vi "电导率电极校准.vi"() -> ()   [LabVIEW 2016, in "斯坦道多参数.lvlib"]
uses:
  <vilib>/Utility/miscctls.llb/LVPointTypeDef.ctl
  <vilib>/Analysis/NI_AALBase.lvlib
panel:
  out "滤波设定":dbl
  in  "刷新按钮":bool
  out "第二点信号值":dbl
  out "第一点信号值":dbl
  out "通讯状态":string
  out "盐度":dbl caption="盐度测量值" format="%#.2f"
  out "温度":dbl format="%#.2f"
  out "当前信号值":dbl caption="信号值" format="%#.2f"
  in  "校准停止":bool
  in  "校准启动":bool
  out "波形图表":sgl(graph) caption="历史曲线"
  out "第二点校准值":dbl
  out "第一点校准值":dbl
  in  "校准模式":u16(ring)=1 items=["两点校准", "单点校准"]
  out "提示":string
  out "最小值":sgl format="%#.2f"
  out "最大值":sgl format="%#.2f"
  out "mean":dbl caption="均值" format="%#.2f"
  out "standard deviation":dbl caption="标准差" format="%#.2f"
  out "变异系数":dbl format="%#.6f"
  out "标液2":dbl
  out "标液1":dbl
  out "当前读取值":dbl caption="测量值" format="%#.2f"
  out "电极系数":dbl format="%#.6f"
  out "偏移值补偿":dbl caption="电导率偏移修正值" format="%#.2f"
  out "温度补偿系数":dbl format="%#.6f"
  # "电导率电极设定"
  # "ppt"
  # "请选择校准模式:"
  # "℃"
  # "μS/cm"
  # "cm"
  # "-1"
  # "%"
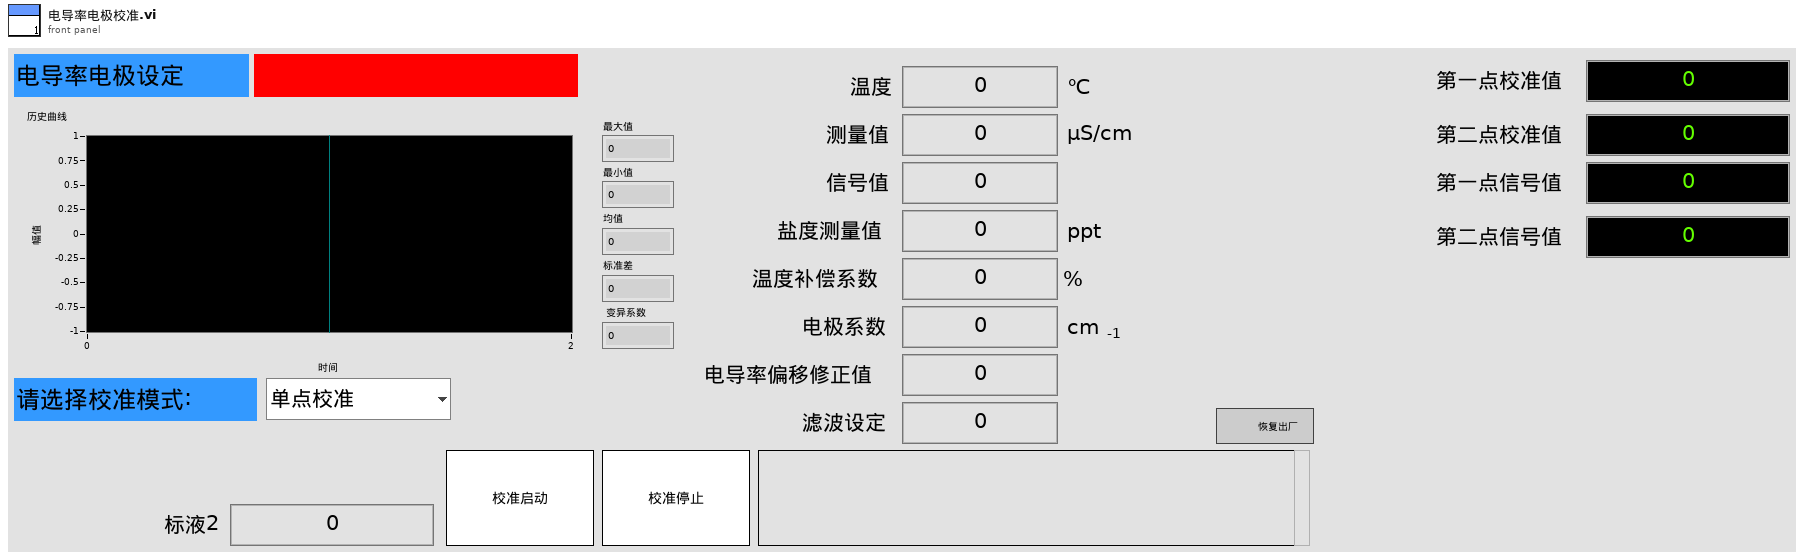
[diagram p1: front panel]
types:
  T1 = enum16{"pH", "DO", "Cond", "Turb", "ORP", "叶绿素a", "藻密度"}
  T2 = typedef "LVPointTypeDef.ctl" = cluster{"Horizontal":i16, "Vertical":i16}
  T3 = cluster{"电极状态标志":u16, "电极型号标志":u16, "电导率测量值":sgl, "温度测量值":sgl, "电导率信号值":sgl, "温度信号值":sgl, "温度补偿系数":sgl, "电导率偏移修正值":sgl, "温度偏移修正值":sgl, "手动温度补偿值":sgl, "电导率电极零点":sgl, "电导率电极斜率":sgl, "命令滤波设定":u16, "温度模式":enum16{"ATC", "MTC"}, "生产批次":u16, "电极序号":u16, "串口地址":u16, "串口波特率":enum16{"9600", "19200", "115200"}, "串口校验位":enum16{"NONE", "ODD", "EVEN"}, "串口停止位":enum16{"1bit", "2bit"}, "第一点标准值":sgl, "第二点标准值":sgl}
  T4 = enum8{"Enabled", "Disabled", "Disabled and Grayed Out"}
  T5 = cluster{"测量量程":dbl, "测量精度":dbl, "测量间隔":dbl, "消解温度":dbl, "消解时长":dbl, "空白校准时间":timestamp, "曲线截距":dbl, "曲线斜率":dbl, "测量检出限":dbl, "测量信号值":dbl, "线性相关系数":dbl, "二次多项式系数":dbl, "标样校准时间":timestamp, "稀释倍数":dbl, "三项式系数":dbl, "空白标定系数":dbl, "量程系数":dbl, "F0/ORPA":dbl, "F1/ORPB":dbl, "F2/ORPK":dbl, "F3":dbl, "F4":dbl, "F5":dbl, "F6":dbl, "F7":dbl, "X0/滴定数":dbl, "量程":dbl}
  T6 = cluster{"ph":bool, "DO":bool, "Cond":bool, "Turb":bool, "叶绿素a":bool, "藻密度":bool, "ORP":bool, "COD":bool}
  T7 = cluster{"温度测量值":sgl, "测量值":sgl, "温度偏移修正值":sgl, "信号值":sgl}
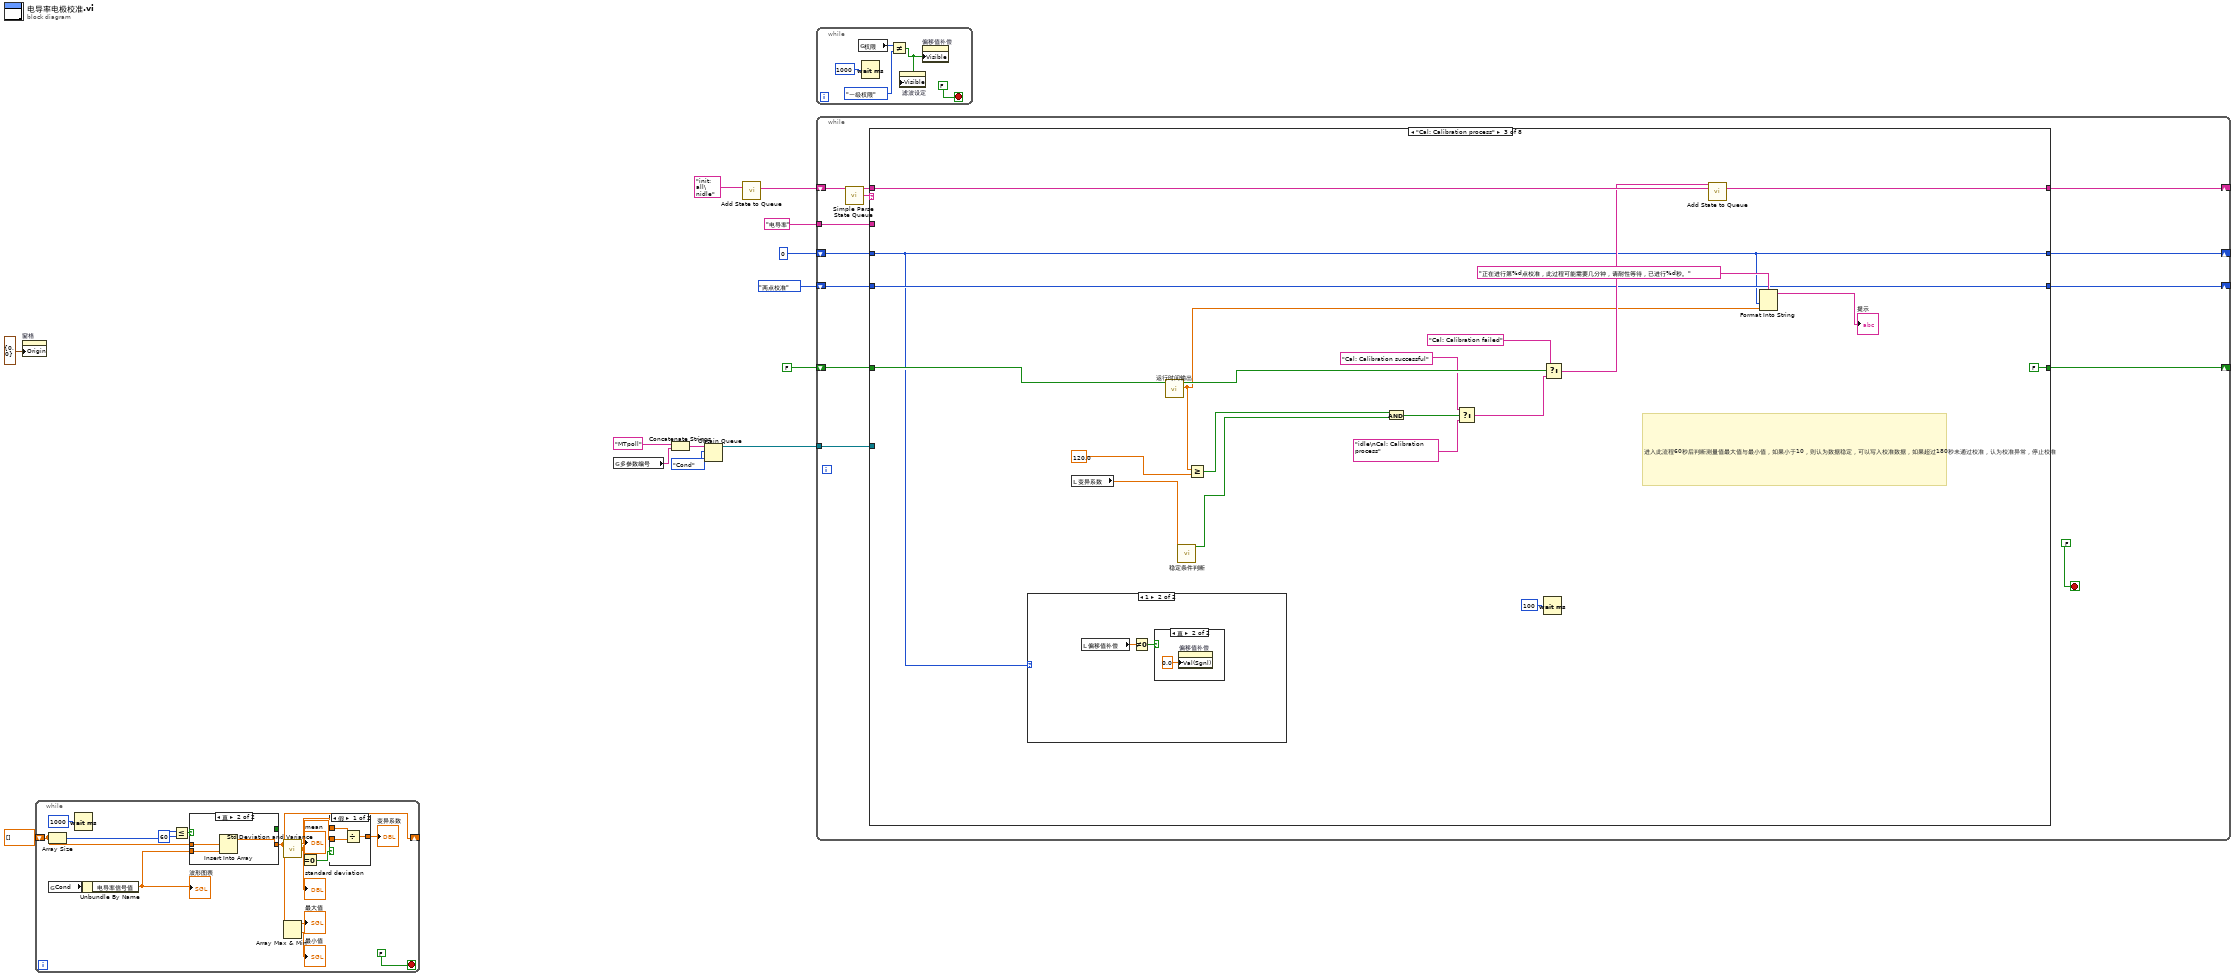
[diagram p0: block diagram]
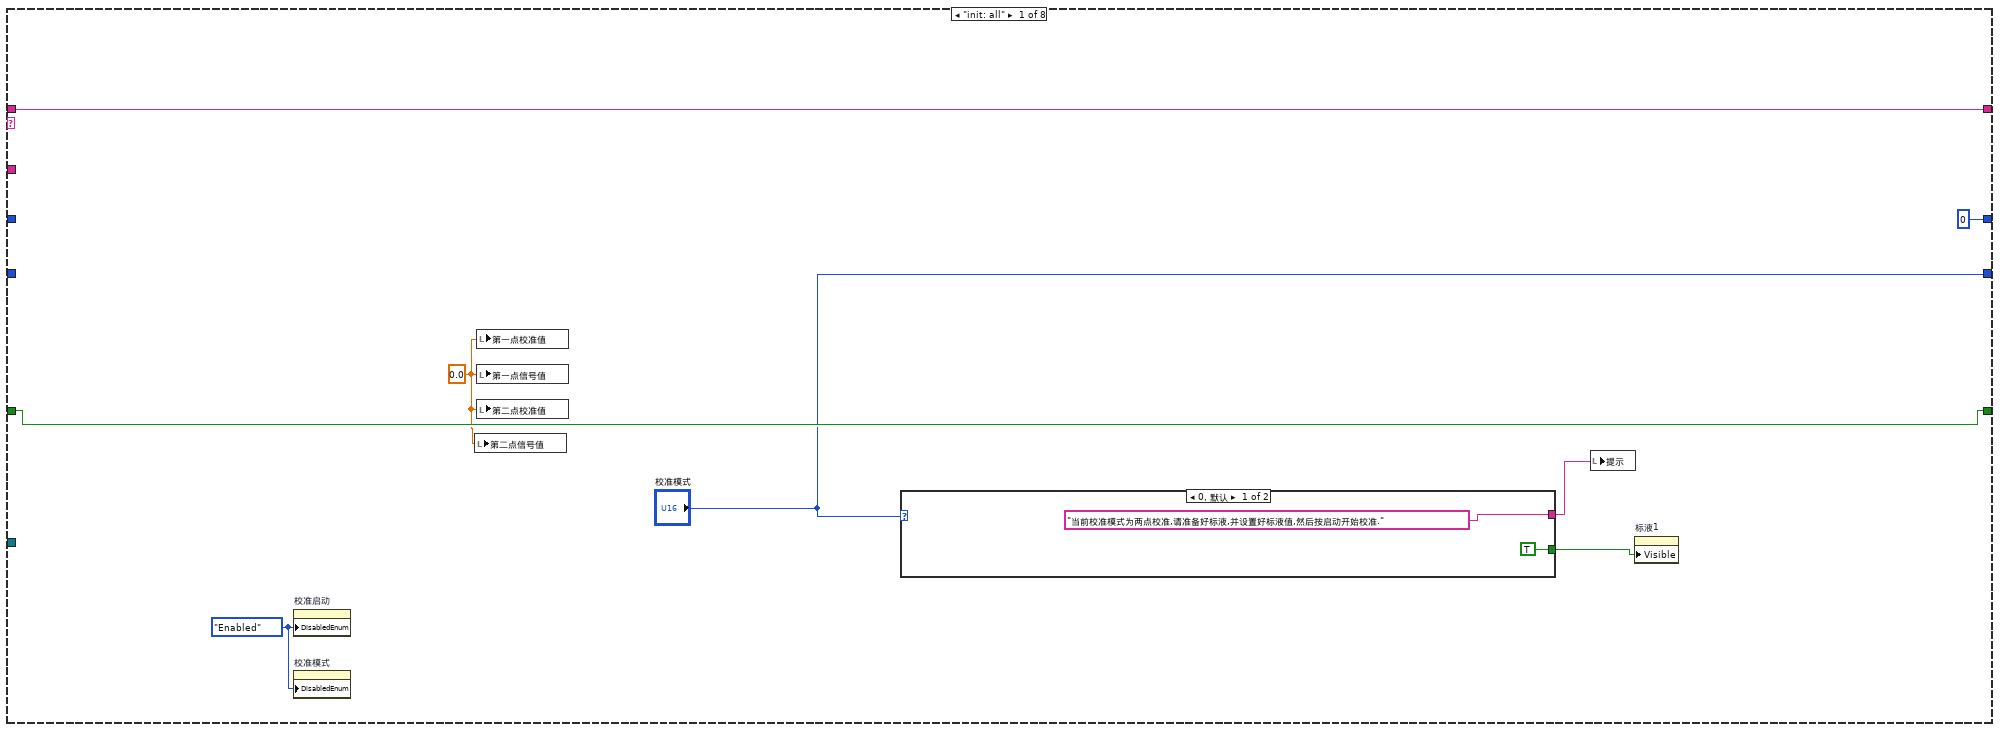
[diagram p2: hidden frame]
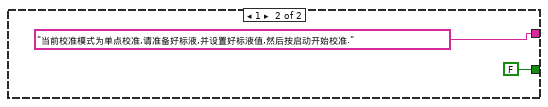
[diagram p3: hidden frame]
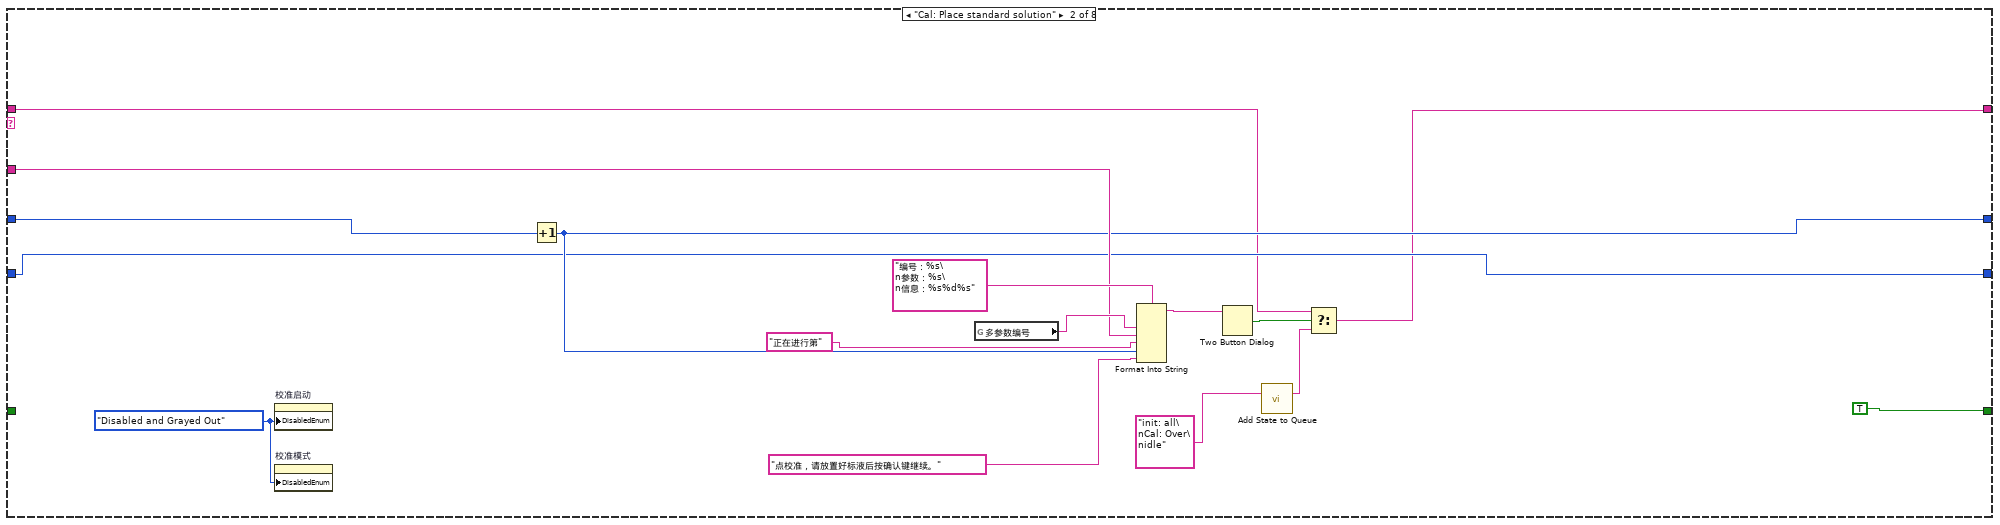
[diagram p4: hidden frame]
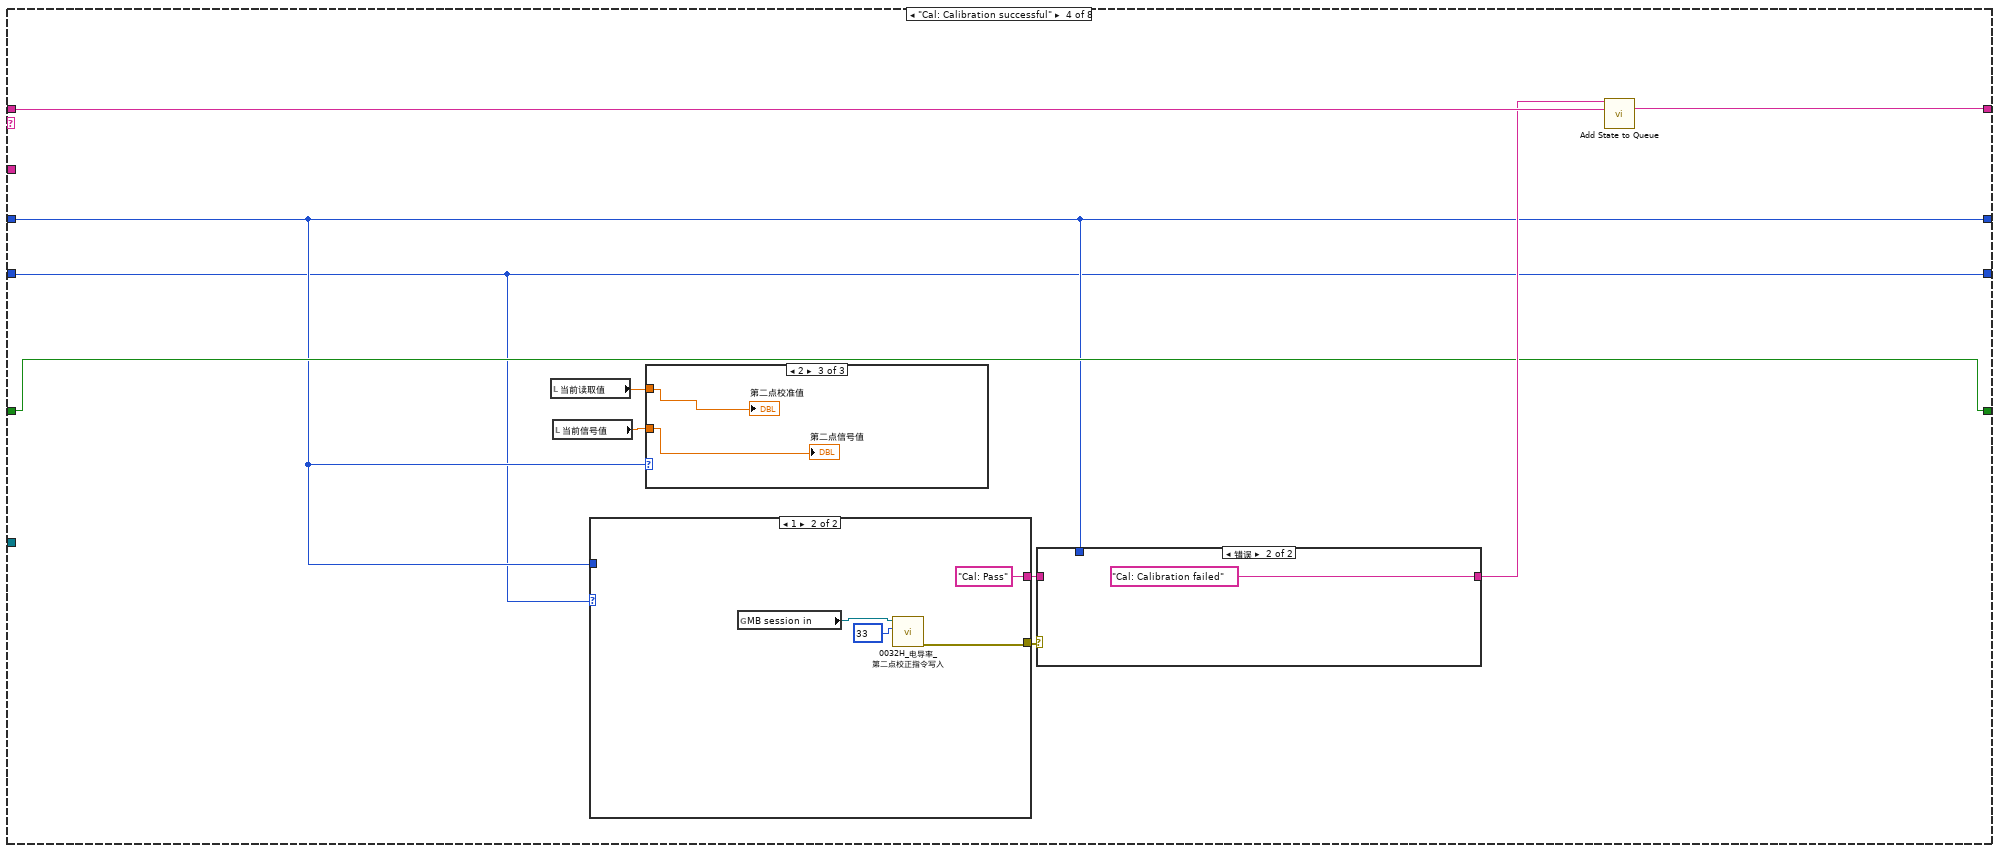
[diagram p7: hidden frame]
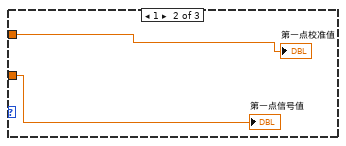
[diagram p9: hidden frame]
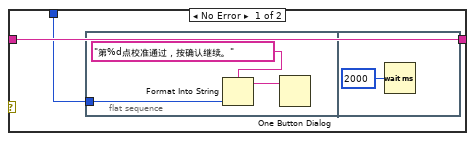
[diagram p10: hidden frame]
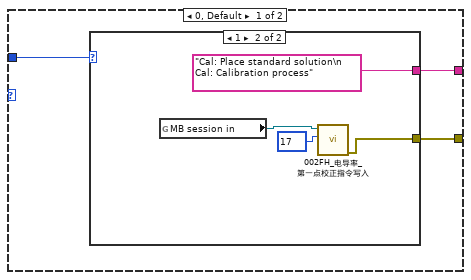
[diagram p11: hidden frame]
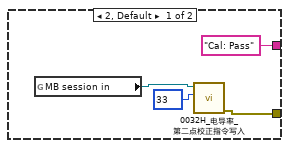
[diagram p12: hidden frame]
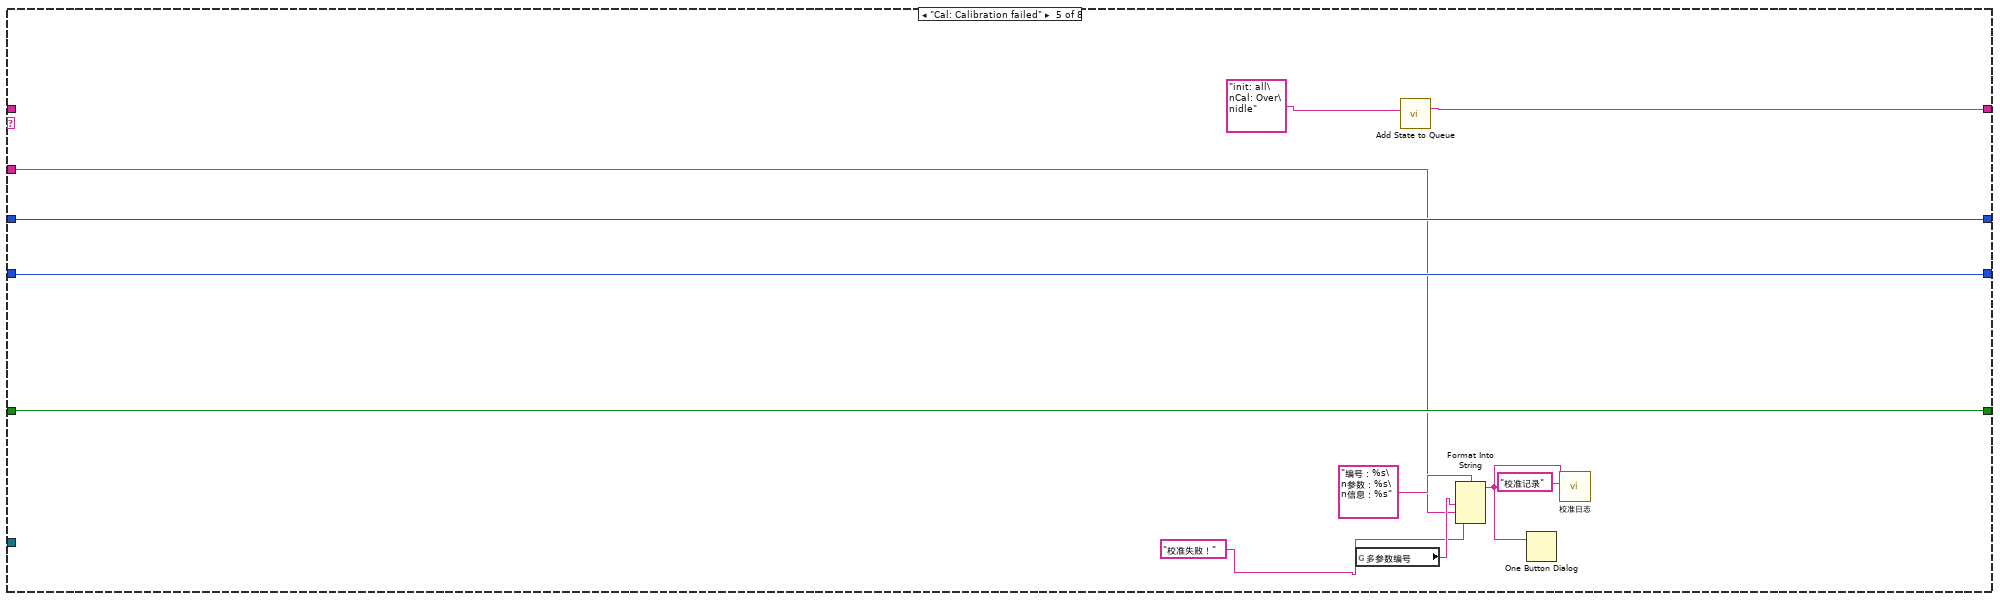
[diagram p13: hidden frame]
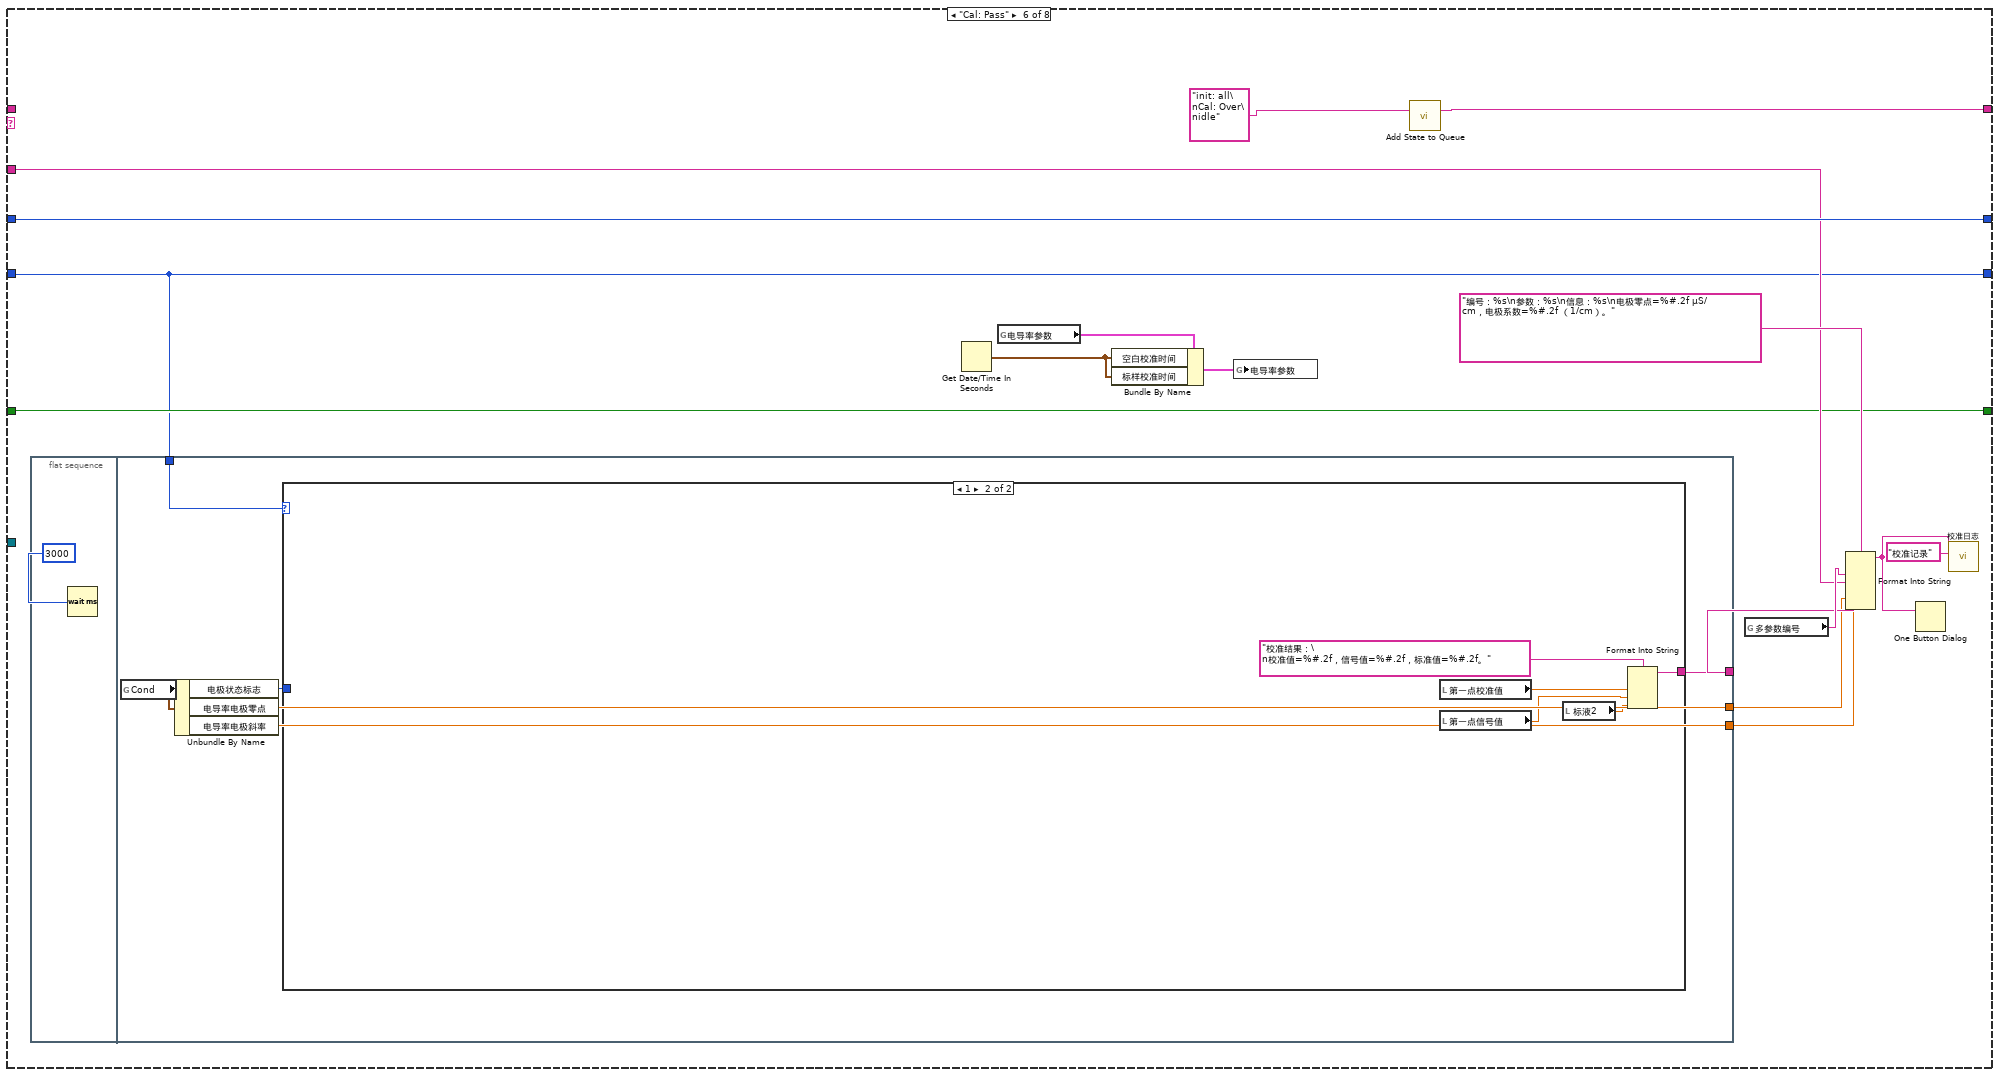
[diagram p14: hidden frame]
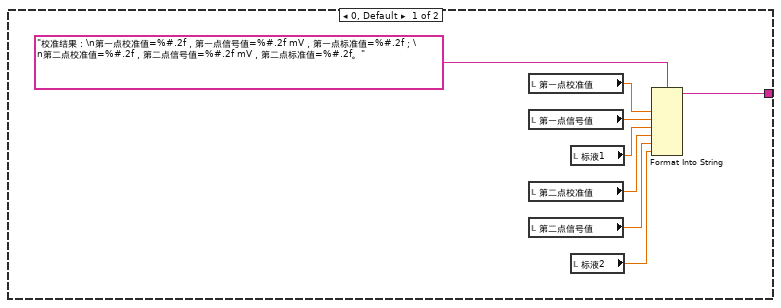
[diagram p15: hidden frame]
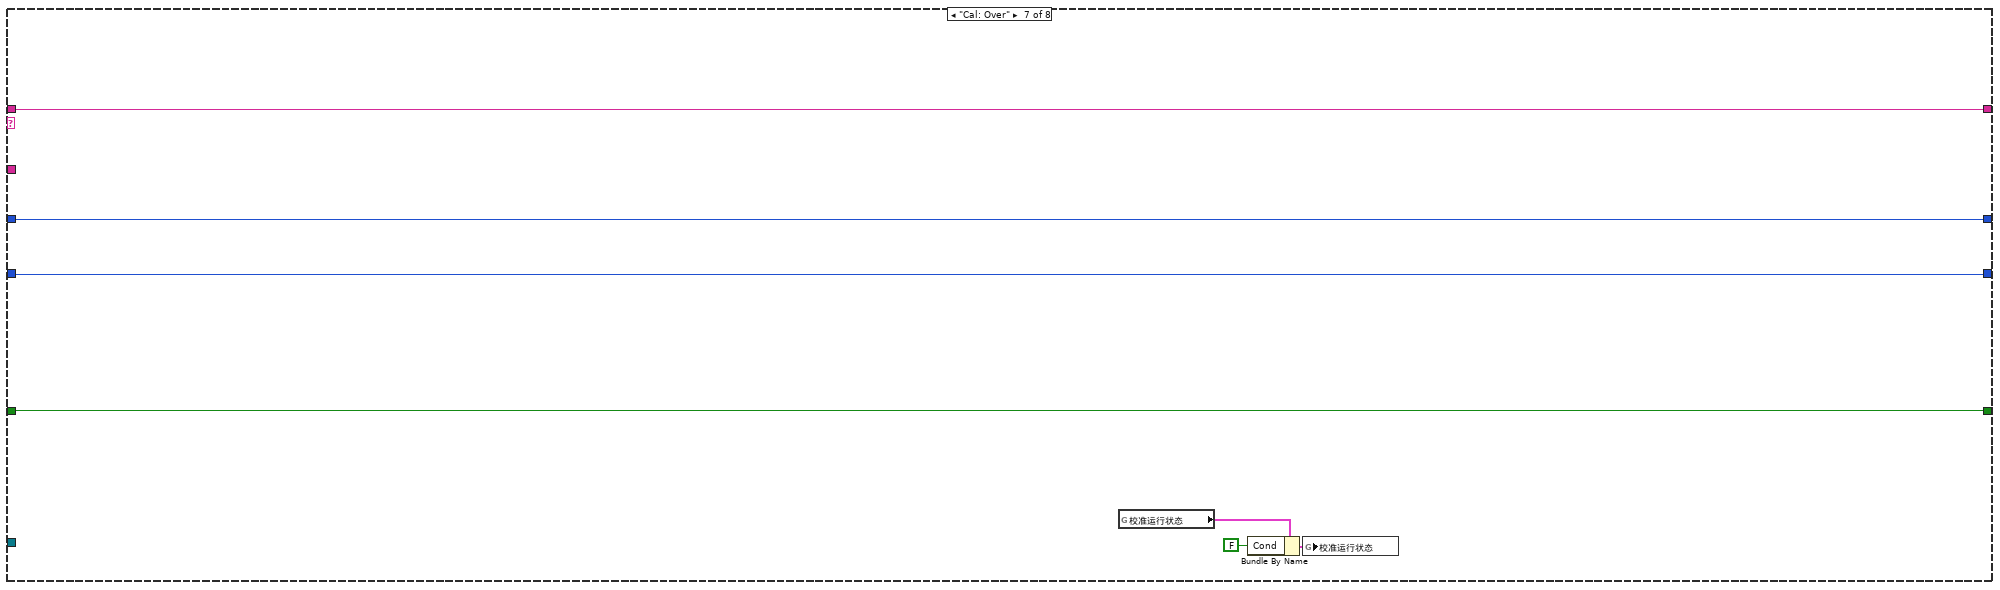
[diagram p16: hidden frame]
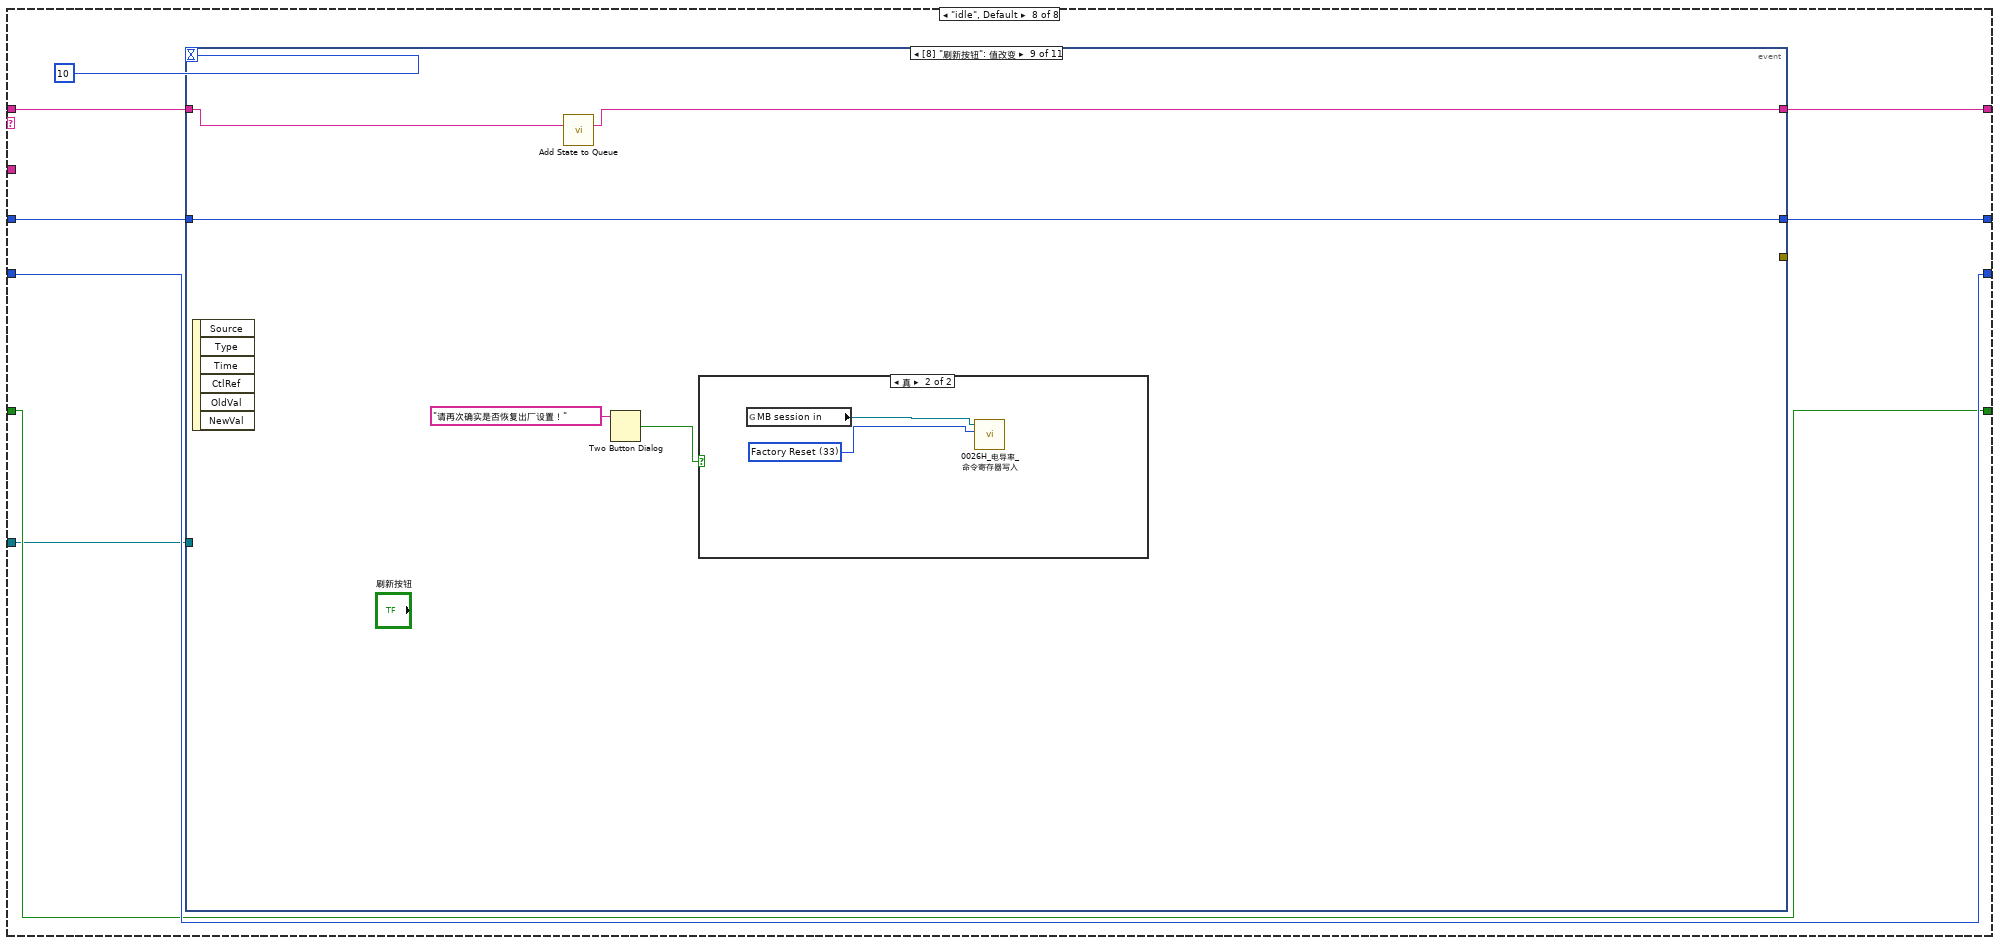
[diagram p17: hidden frame]
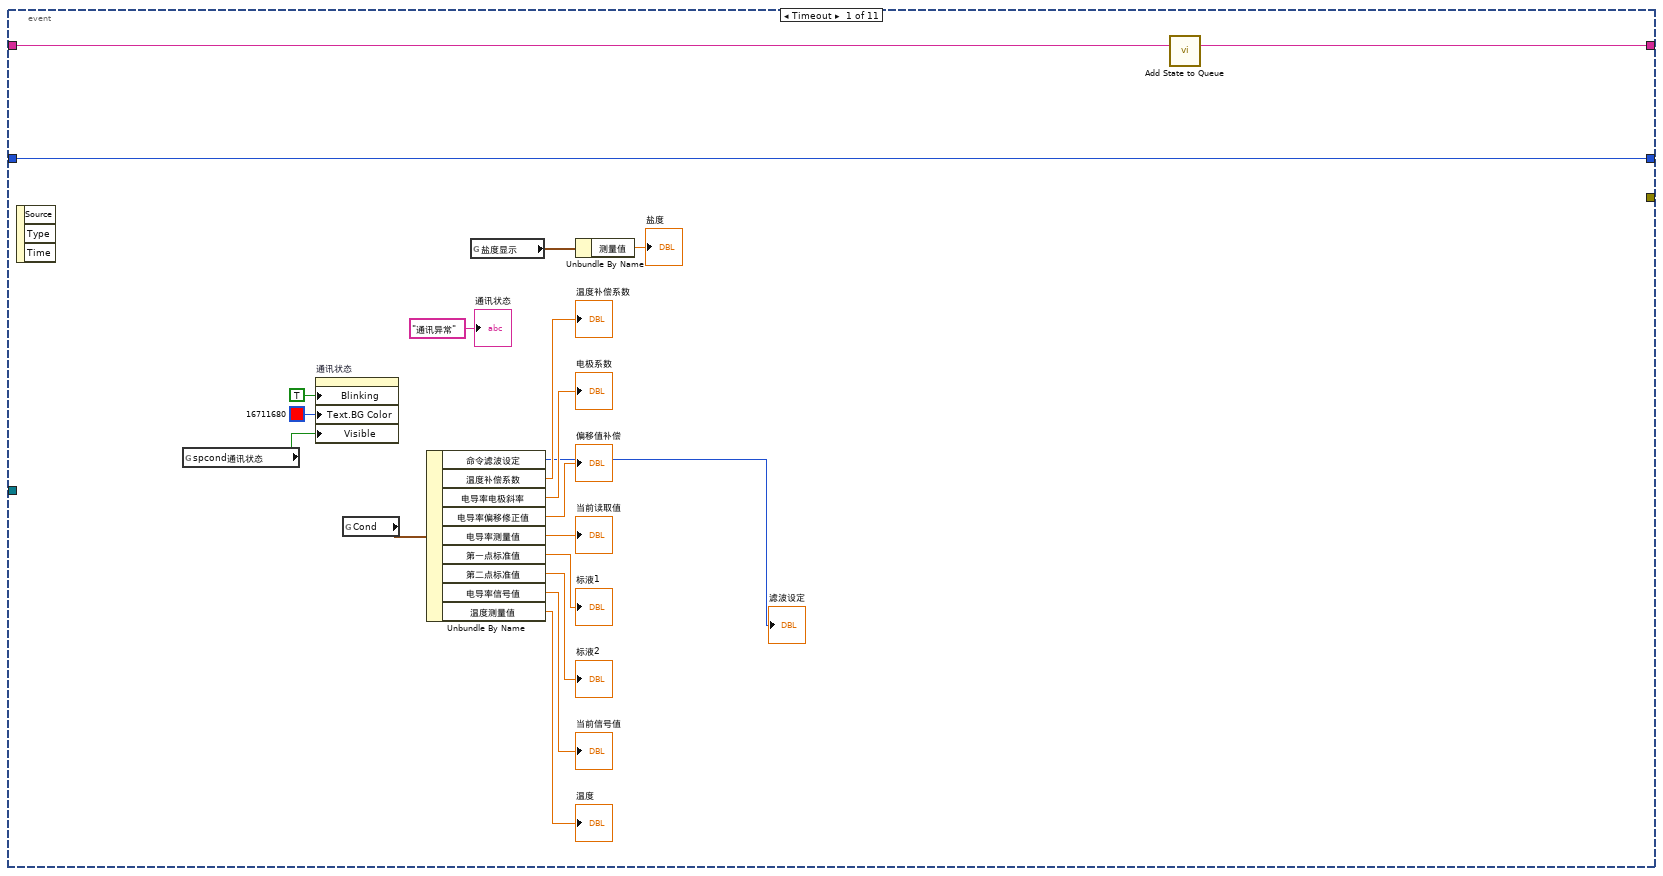
[diagram p18: hidden frame]
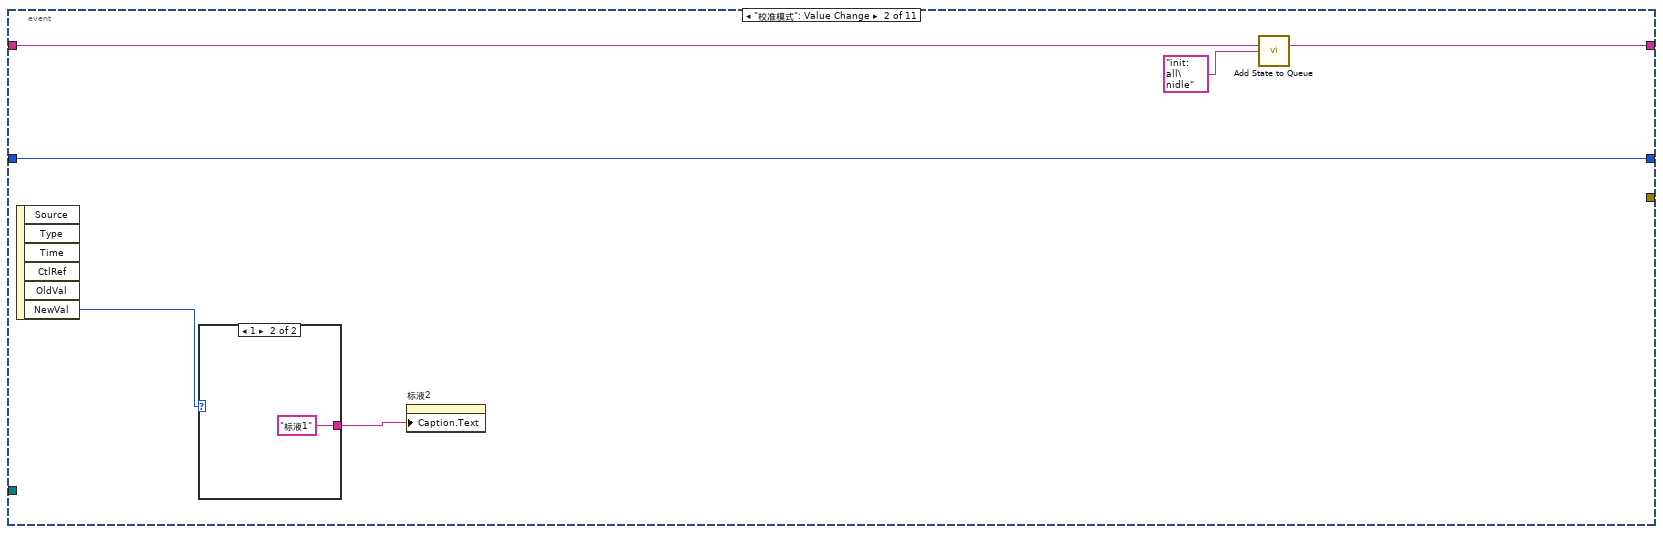
[diagram p19: hidden frame]
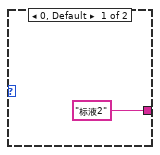
[diagram p20: hidden frame]
diagram:
  n1 = property on="窗格" class="Pane"("Origin"=T2 {"Horizontal"=0, "Vertical"=0} ("原点")) -> ()  [unwired: 2 in, 2 out]
  n2 = while {
    shift-right: [w17] -> _
    shift-left: sgl[] [] -> [w24]
    stop <- FALSE stop-if-true
    n3 = Array Size(array=w24) -> (size(s)=w26:i32)
    n4 = global read "国弘过程全局变量.vi" "Cond"() -> (w18:T3)
    n5 = Wait (ms)(milliseconds to wait=u32 1000 ("等待时间（毫秒）")) -> ()  [unwired: 1 out]
    n6 = Unbundle By Name(w18) -> ("电导率信号值"=w14:sgl)
    "波形图表" <- w14
    n7 = Less Or Equal?(x=w26, y=60) -> (x <= y?=w25:bool)
    n8 = case shown="真" w25 {
      tunnel: w24 -> [w37 w40]
      tunnel: w14 -> [w35 w39]
      tunnel: [w33 w38] -> w17
      tunnel: [TRUE _] -> _
      frame False {
        n9 = Replace Array Subset(array=w37, new element=w35) -> (w36:sgl[])  [unwired: 1 in]
        n10 = Rotate 1D Array(1:w36, 2:-1 ("n")) -> (0:w33:sgl[])
      }
      frame True {
        n11 = Insert Into Array(array=w40, new element=w39) -> (w38:sgl[])  [unwired: 1 in]
      }
    }
    n12 = call <vilib>:"Std Deviation and Variance.vi"("X"=w17) -> ("mean"=w22:dbl, "standard deviation"=w21:dbl)  [unwired: 1 in, 1 out]
    "mean" <- w22
    "standard deviation" <- w21
    n13 = Array Max & Min(array=w17) -> (max value=→"最大值":sgl, min value=→"最小值":sgl)  [unwired: 2 out]
    n14 = Equal To 0?(x=w22) -> (x = 0?=w23:bool)
    n15 = case shown="假" w23 {
      tunnel: w21 -> [w31 _]
      tunnel: [w30 _] -> w20
      tunnel: w22 -> [w29 _]
      frame False {
        n16 = Divide(x=w31, y=w29) -> (x/y=w30:dbl)
      }
      frame True {
      }
    }
    "变异系数" <- w20
  }
  n17 = global read "多参数全局变量.vi" "多参数编号"() -> (w2:string)
  n18 = Concatenate Strings("MTpoll" ("名称（未命名）"), w2) -> (w4:string)
  n19 = Obtain Queue(name (unnamed)=w4, element data type=T1."Cond" ("枚举")) -> (queue out=w1:refnum<queue>)  [unwired: 3 in, 2 out]
  n20 = call "Add State to Queue.vi"("State(s) In (\"\")"="init: all\nidle" ("State(s) In (\"\")")) -> ("States Out"=w10:string)  [unwired: 14 in]
  n21 = while {
    stop <- FALSE stop-if-true
    n22 = global read "多参数全局变量.vi" "权限"() -> (w44:enum16{"一级权限", "二级权限", "三级权限"})
    n23 = Wait (ms)(milliseconds to wait=u32 1000 ("等待时间（毫秒）")) -> ()  [unwired: 1 out]
    n24 = Not Equal?(x=w44, y=enum16{"一级权限", "二级权限", "三级权限"}."一级权限") -> (x != y?=w41:bool)
    n25 = property on="滤波设定" class="DigNum (严格)"("Visible"=w41) -> ()  [unwired: 2 in, 2 out]
    n26 = property on="偏移值补偿" class="DigNum (严格)"("Visible"=w41) -> ()  [unwired: 2 in, 2 out]
  }
  n27 = while {
    shift-right: [w54] -> _
    shift-left: w10 -> [w58]
    shift-right: [w51] -> _
    shift-left: 0 -> [w53]
    tunnel: "电导率" ("State(s) In (\"\")") -> [w52]
    shift-right: [w49] -> _
    shift-left: enum16{"两点校准", "单点校准"}."两点校准" ("校准模式") -> [w50]
    shift-right: [w47] -> _
    shift-left: FALSE -> [w48]
    tunnel: w1 -> [w46]
    stop <- FALSE stop-if-true
    n28 = call "Simple Parse State Queue.vi"("State Queue"=w58) -> ("Remain States"=w55:string, "Next State"=w56:string)  [unwired: 13 in]
    n29 = case shown="\"Cal: Calibration process\"" w56 {
      tunnel: w55 -> [w66 w74 w106 w118 _ _ w200 w208]
      tunnel: [w66 w73 w105 w117 w154 w164 w200 w207] -> w54
      tunnel: w53 -> [_ w82 w91 w112 w157 w173 w199 w205]
      tunnel: w52 -> [_ w83 _ _ w148 w169 _ _]
      tunnel: [0 w80 w91 w112 w157 w173 w199 w206] -> w51
      tunnel: w50 -> [_ w79 w92 w111 w156 w165 w198 w204]
      tunnel: ["校准模式" w79 w92 w111 w156 w165 w198 w204] -> w49
      tunnel: w48 -> [w63 _ w94 w113 w155 w168 w197 w202]
      tunnel: [w63 TRUE FALSE w113 w155 w168 w197 w202] -> w47
      tunnel: w46 -> [_ _ _ _ _ _ _ w201]
      frame "init: all" {
        w61 = T4."Enabled" ("禁用")
        w60 = 0.0 ("第一点校准值")
        n30 = property on="校准启动" class="Bool"("DisabledEnum"=w61) -> ()  [unwired: 2 in, 2 out]
        n31 = property on="校准模式" class="Ring (严格)"("DisabledEnum"=w61) -> ()  [unwired: 2 in, 2 out]
        n32 = local write "第二点信号值"(w60) -> ()
        n33 = local write "第一点校准值"(w60) -> ()
        n34 = local write "第一点信号值"(w60) -> ()
        n35 = local write "第二点校准值"(w60) -> ()
        n36 = case shown="0, 默认" "校准模式" {
          tunnel: ["当前校准模式为两点校准,请准备好标液,并设置好标液值,然后按启动开始校准." ("提示") "当前校准模式为单点校准,请准备好标液,并设置好标液值,然后按启动开始校准." ("提示")] -> w65
          tunnel: [TRUE ("可见") FALSE ("可见")] -> w59
          frame 0, Default {
          }
          frame 1 {
          }
        }
        n37 = local write "提示"(w65) -> ()
        n38 = property on="标液1" class="DigNum (严格)"("Visible"=w59) -> ()  [unwired: 2 in, 2 out]
      }
      frame "Cal: Place standard solution" {
        w72 = T4."Disabled and Grayed Out" ("禁用")
        n39 = property on="校准启动" class="Bool"("DisabledEnum"=w72) -> ()  [unwired: 2 in, 2 out]
        n40 = property on="校准模式" class="Ring (严格)"("DisabledEnum"=w72) -> ()  [unwired: 2 in, 2 out]
        n41 = Increment(x=w82) -> (x+1=w80:i32)
        n42 = global read "多参数全局变量.vi" "多参数编号"() -> (w85:string)
        n43 = Format Into String(format string="编号：%s\n参数：%s\n信息：%s%d%s" ("格式字符串"), w85, w83, "正在进行第" ("消息"), w80, "点校准，请放置好标液后按确认键继续。" ("消息")) -> (resulting string=w77:string)  [unwired: 2 in, 1 out]
        n44 = Two Button Dialog(message=w77) -> (T button?=w76:bool)  [unwired: 2 in]
        n45 = call "Add State to Queue.vi"("State(s) In (\"\")"="init: all\nCal: Over\nidle" ("State(s) In (\"\")")) -> ("States Out"=w75:string)  [unwired: 14 in]
        n46 = Select(t=w74, s=w76, f=w75) -> (s? t:f=w73:string)
      }
      frame "Cal: Calibration process" {
        # "进入此流程60秒后判断测量值最大值与最小值，如果小于10，则认为数据稳定，可以写入校准数据，如果超过180秒未通过校准，认为校准异常，停止校准"
        n47 = case shown="1" w91 {
          frame 0, Default {
          }
          frame 1 {
            n48 = local read "偏移值补偿"() -> (w108:dbl)
            n49 = Not Equal To 0?(x=w108) -> (x != 0?=w109:bool)
            n50 = case shown="真" w109 {
              frame False {
              }
              frame True {
                n51 = property on="偏移值补偿" class="DigNum (严格)"("Val(Sgnl)"=0.0 ("值(信号)")) -> ()  [unwired: 2 in, 2 out]
              }
            }
          }
        }
        n52 = local read "变异系数"() -> (w88:dbl)
        n53 = call "运行时间输出.vi"("初始化"=w94) -> ("Elapsed Time (s)"=w90:dbl, "Time has Elapsed"=w107:bool)  [unwired: 9 in]
        n54 = call "稳定条件判断.vi"("变异系数"=w88) -> ("布尔"=w87:bool)  [unwired: 10 in]
        n55 = Greater Or Equal?(x=w90, y=120.0) -> (x >= y?=w102:bool)
        n56 = And(x=w102, y=w87) -> (x .and. y?=w99:bool)
        n57 = Select(t="Cal: Calibration successful" ("State(s) In (\"\")"), s=w99, f="idle\nCal: Calibration process" ("State(s) In (\"\")")) -> (s? t:f=w98:string)
        n58 = Wait (ms)(milliseconds to wait=u32 100 ("等待时间（毫秒）")) -> ()  [unwired: 1 out]
        n59 = Select(t="Cal: Calibration failed" ("State(s) In (\"\")"), s=w107, f=w98) -> (s? t:f=w97:string)
        n60 = call "Add State to Queue.vi"("State(s) In Front (\"\")"=w97, "State(s) In (\"\")"=w106) -> ("States Out"=w105:string)  [unwired: 13 in]
        n61 = Format Into String(format string="正在进行第%d点校准，此过程可能需要几分钟，请耐性等待，已进行%d秒。" ("格式字符串"), w91, w90) -> (resulting string=→"提示":string)  [unwired: 2 in, 1 out]
      }
      frame "Cal: Calibration successful" {
        n62 = local read "当前读取值"() -> (w114:dbl)
        n63 = local read "当前信号值"() -> (w115:dbl)
        n64 = case shown="1" w111 {
          tunnel: [w134 w143] -> w120
          tunnel: [w133 "Cal: Pass" ("State(s) In (\"\")")] -> w119
          tunnel: w112 -> [w132 _]
          frame 0, Default {
            n65 = case shown="1" w132 {
              tunnel: [w135 w139] -> w134
              tunnel: ["Cal: Pass" ("State(s) In (\"\")") "Cal: Place standard solution\n Cal: Calibration process" ("State(s) In (\"\")")] -> w133
              frame 2, Default {
                n66 = global read "多参数全局变量.vi" "MB session in"() -> (w137:refnum<class "MB_Master.lvclass">)
                n67 = call "0032H_电导率_第二点校正指令写入.vi"("数值"=u16 33, "MB session in"=w137) -> ("error out"=w135:errorcluster)  [unwired: 8 in, 1 out]
              }
              frame 1 {
                n68 = global read "多参数全局变量.vi" "MB session in"() -> (w141:refnum<class "MB_Master.lvclass">)
                n69 = call "002FH_电导率_第一点校正指令写入.vi"("数值"=u16 17, "MB session in"=w141) -> ("error out"=w139:errorcluster)  [unwired: 8 in, 1 out]
              }
            }
          }
          frame 1 {
            n70 = global read "多参数全局变量.vi" "MB session in"() -> (w145:refnum<class "MB_Master.lvclass">)
            n71 = call "0032H_电导率_第二点校正指令写入.vi"("数值"=u16 33, "MB session in"=w145) -> ("error out"=w143:errorcluster)  [unwired: 8 in, 1 out]
          }
        }
        n72 = case shown="2" w112 {
          tunnel: w115 -> [_ w122 w124]
          tunnel: w114 -> [_ w121 w123]
          frame 0, Default {
          }
          frame 1 {
            "第一点信号值" <- w122
            "第一点校准值" <- w121
          }
          frame 2 {
            "第二点信号值" <- w124
            "第二点校准值" <- w123
          }
        }
        n73 = case shown="错误" w120 {
          tunnel: w119 -> [w126 _]
          tunnel: [w126 "Cal: Calibration failed" ("State(s) In (\"\")")] -> w116
          tunnel: w112 -> [w125 _]
          frame No Error {
            n74 = flat-sequence {
              tunnel: w125 -> [w127]
              frame #0 {
                n75 = Format Into String(format string="第%d点校准通过，按确认继续。" ("格式字符串"), w127) -> (resulting string=w129:string)  [unwired: 2 in, 1 out]
                n76 = One Button Dialog(message=w129) -> ()  [unwired: 1 in, 1 out]
              }
              frame #1 {
                n77 = Wait (ms)(milliseconds to wait=u32 2000 ("等待时间（毫秒）")) -> ()  [unwired: 1 out]
              }
            }
          }
          frame Error {
          }
        }
        n78 = call "Add State to Queue.vi"("State(s) In Front (\"\")"=w116, "State(s) In (\"\")"=w118) -> ("States Out"=w117:string)  [unwired: 13 in]
      }
      frame "Cal: Calibration failed" {
        n79 = global read "多参数全局变量.vi" "多参数编号"() -> (w151:string)
        n80 = call "Add State to Queue.vi"("State(s) In (\"\")"="init: all\nCal: Over\nidle" ("State(s) In (\"\")")) -> ("States Out"=w154:string)  [unwired: 14 in]
        n81 = Format Into String(format string="编号：%s\n参数：%s\n信息：%s" ("格式字符串"), w151, w148, "校准失败！" ("消息")) -> (resulting string=w150:string)  [unwired: 2 in, 1 out]
        n82 = One Button Dialog(message=w150) -> ()  [unwired: 1 in, 1 out]
        n83 = call "校准日志.vi"("table"="校准记录", "日志信息"=w150) -> ()  [unwired: 9 in, 1 out]
      }
      frame "Cal: Pass" {
        n84 = flat-sequence {
          tunnel: [w178] -> w166
          tunnel: w165 -> [w177]
          tunnel: [w176] -> w163
          tunnel: [w175] -> w162
          frame #0 {
            n85 = Wait (ms)(milliseconds to wait=u32 3000 ("等待时间（毫秒）")) -> ()  [unwired: 1 out]
          }
          frame #1 {
            n86 = global read "国弘过程全局变量.vi" "Cond"() -> (w179:T3)
            n87 = Unbundle By Name(w179) -> ("电极状态标志"=w180:u16, "电导率电极零点"=w176:sgl, "电导率电极斜率"=w175:sgl)
            n88 = case shown="1" w177 {
              tunnel: [w188 w193] -> w178
              tunnel: w180 -> [_ _]
              frame 0, Default {
                n89 = local read "第一点校准值"() -> (w186:dbl)
                n90 = local read "第一点信号值"() -> (w187:dbl)
                n91 = local read "第二点校准值"() -> (w183:dbl)
                n92 = local read "第二点信号值"() -> (w182:dbl)
                n93 = local read "标液1"() -> (w184:dbl)
                n94 = local read "标液2"() -> (w181:dbl)
                n95 = Format Into String(format string="校准结果：\n第一点校准值=%#.2f，第一点信号值=%#.2f mV，第一点标准值=%#.2f；\n第二点校准值=%#.2f，第二点信号值=%#.2f mV，第二点标准值=%#.2f。" ("提示"), w186, w187, w184, w183, w182, w181) -> (resulting string=w188:string)  [unwired: 2 in, 1 out]
              }
              frame 1 {
                n96 = local read "第一点校准值"() -> (w192:dbl)
                n97 = local read "第一点信号值"() -> (w190:dbl)
                n98 = local read "标液2"() -> (w189:dbl)
                n99 = Format Into String(format string="校准结果：\n校准值=%#.2f，信号值=%#.2f，标准值=%#.2f。" ("提示"), w192, w190, w189) -> (resulting string=w193:string)  [unwired: 2 in, 1 out]
              }
            }
          }
        }
        n100 = Get Date/Time In Seconds() -> (seconds since 1Jan1904=w158:timestamp)
        n101 = global read "断电保存变量.vi" "电导率参数"() -> (w160:T5)
        n102 = Bundle By Name(cluster=w160, "空白校准时间"=w158, "标样校准时间"=w158) -> (w159:T5)
        n103 = global write "断电保存变量.vi" "电导率参数"(w159) -> ()
        n104 = call "Add State to Queue.vi"("State(s) In (\"\")"="init: all\nCal: Over\nidle" ("State(s) In (\"\")")) -> ("States Out"=w164:string)  [unwired: 14 in]
        n105 = global read "多参数全局变量.vi" "多参数编号"() -> (w170:string)
        n106 = Format Into String(format string="编号：%s\n参数：%s\n信息：%s\n电极零点=%#.2f μS/cm，电极系数=%#.2f （1/cm）。" ("格式字符串"), w170, w169, w166, w163, w162) -> (resulting string=w167:string)  [unwired: 2 in, 1 out]
        n107 = One Button Dialog(message=w167) -> ()  [unwired: 1 in, 1 out]
        n108 = call "校准日志.vi"("table"="校准记录", "日志信息"=w167) -> ()  [unwired: 9 in, 1 out]
      }
      frame "Cal: Over" {
        n109 = global read "多参数全局变量.vi" "校准运行状态"() -> (w195:T6)
        n110 = Bundle By Name(cluster=w195, "Cond"=FALSE) -> (w196:T6)
        n111 = global write "多参数全局变量.vi" "校准运行状态"(w196) -> ()
      }
      frame "idle", Default {
        n112 = event shown="[8] \"刷新按钮\": 值改变" {
          selector: _ -> [_ _ _ _ _ _ _ _ _ _ _]
          dyn-events: _ -> [_ _ _ _ _ _ _ _ _ _ _]
          timeout: 10 -> [_ _ _ _ _ _ _ _ _ _ _]
          tunnel: [_ _ _ w245 w254 w263 w272 w281 _ _ _] -> _
          tunnel: w208 -> [w227 w233 w240 w246 w258 w264 w278 w287 w292 w301 _]
          tunnel: [w226 w232 w241 w250 w259 w265 w277 w286 w291 w300 w303] -> w207
          tunnel: [w225 w230 w242 w251 w260 w266 w276 w285 w290 w298 w304] -> w206
          tunnel: w205 -> [w225 w230 w242 w251 w260 w266 w276 w285 w290 w298 w304]
          tunnel: w201 -> [_ _ _ w244 w253 w262 w271 w280 _ _ _]
          event Timeout {
            n113 = event-data() -> ()  [unwired: 1 in, 3 out]
            n114 = global read "多参数全局变量.vi" "spcond通讯状态"() -> (w223:bool)
            n115 = property on="通讯状态" class="Str"("Blinking"=TRUE ("闪烁"), "Text.BG Color"=u32 16711680, "Visible"=w223) -> ()  [unwired: 2 in, 2 out]
            n116 = global read "国弘过程全局变量.vi" "Cond"() -> (w210:T3)
            n117 = Unbundle By Name(w210) -> ("命令滤波设定"=→"滤波设定":u16, "温度补偿系数"=→"温度补偿系数":sgl, "电导率电极斜率"=→"电极系数":sgl, "电导率偏移修正值"=→"偏移值补偿":sgl, "电导率测量值"=→"当前读取值":sgl, "第一点标准值"=→"标液1":sgl, "第二点标准值"=→"标液2":sgl, "电导率信号值"=→"当前信号值":sgl, "温度测量值"=→"温度":sgl)
            n118 = global read "多参数全局变量.vi" "盐度显示"() -> (w219:T7)
            n119 = Unbundle By Name(w219) -> ("测量值"=→"盐度":sgl)
            n120 = call "Add State to Queue.vi"("State(s) In (\"\")"=w227) -> ("States Out"=w226:string)  [unwired: 14 in]
            "通讯状态" <- "通讯异常" ("当前串口")
          }
          event "校准模式": Value Change {
            n121 = event-data() -> ("NewVal"=w229:u16)  [unwired: 1 in, 5 out]
            n122 = case shown="1" w229 {
              tunnel: ["标液2" ("标题.文本") "标液1" ("标题.文本")] -> w228
              frame 0, Default {
              }
              frame 1 {
              }
            }
            n123 = property on="标液2" class="DigNum (严格)"("Caption.Text"=w228) -> ()  [unwired: 2 in, 2 out]
            n124 = call "Add State to Queue.vi"("State(s) In (\"\")"=w233, "State(s) At Back (\"\")"="init: all\nidle" ("State(s) In (\"\")")) -> ("States Out"=w232:string)  [unwired: 13 in]
          }
          event "标液2", "偏移值补偿", "电极系数", "温度补偿系数", "滤波设定": Mouse Down {
            n125 = event-data() -> ("CtlRef"=w239:refnum<vi>)  [unwired: 1 in, 7 out]
            n126 = property class="DigNum (严格)"(reference=w239) -> (reference out=w236:refnum<vi>, "Value"=w237:dbl)  [unwired: 1 in, 1 out]
            n127 = call "数字键盘.vi"("OldNumber"=w237) -> ("NewNumber"=w238:dbl)  [unwired: 1 in]
            n128 = property class="DigNum (严格)"(reference=w236, "Val(Sgnl)"=w238) -> ()  [unwired: 1 in, 2 out]
            n129 = call "Add State to Queue.vi"("State(s) In (\"\")"=w240) -> ("States Out"=w241:string)  [unwired: 14 in]
          }
          event "标液2": Value Change {
            n130 = event-data() -> ("NewVal"=w248:dbl)  [unwired: 1 in, 5 out]
            n131 = global read "多参数全局变量.vi" "MB session in"() -> (w249:refnum<class "MB_Master.lvclass">)
            n132 = call "0033H_电导率_第二点标准值写入.vi"("数值"=w248, "MB session in"=w249) -> ("error out"=w247:errorcluster)  [unwired: 8 in, 1 out]
            n133 = Enqueue Element At Opposite End(queue=w244, element=T1."Cond" ("元素"), error in (no error)=w247) -> (error out=w245:errorcluster)  [unwired: 1 in, 2 out]
            n134 = call "Add State to Queue.vi"("State(s) In (\"\")"=w246) -> ("States Out"=w250:string)  [unwired: 14 in]
          }
          event "滤波设定": Value Change {
            n135 = event-data() -> ("NewVal"=w256:dbl)  [unwired: 1 in, 5 out]
            n136 = global read "多参数全局变量.vi" "MB session in"() -> (w257:refnum<class "MB_Master.lvclass">)
            n137 = call "0027H_电导率_数位滤波设定写入.vi"("数值"=w256, "MB session in"=w257) -> ("error out"=w255:errorcluster)  [unwired: 8 in, 1 out]
            n138 = Enqueue Element At Opposite End(queue=w253, element=T1."Cond" ("元素"), error in (no error)=w255) -> (error out=w254:errorcluster)  [unwired: 1 in, 2 out]
            n139 = call "Add State to Queue.vi"("State(s) In (\"\")"=w258) -> ("States Out"=w259:string)  [unwired: 14 in]
          }
          event "电极系数": Value Change {
            n140 = event-data() -> ("NewVal"=w268:dbl)  [unwired: 1 in, 5 out]
            n141 = global read "多参数全局变量.vi" "MB session in"() -> (w269:refnum<class "MB_Master.lvclass">)
            n142 = call "0014H_电导率_电极系数写入.vi"("数值"=w268, "MB session in"=w269) -> ("error out"=w267:errorcluster)  [unwired: 8 in, 1 out]
            n143 = Enqueue Element At Opposite End(queue=w262, element=T1."Cond" ("元素"), error in (no error)=w267) -> (error out=w263:errorcluster)  [unwired: 1 in, 2 out]
            n144 = call "Add State to Queue.vi"("State(s) In (\"\")"=w264) -> ("States Out"=w265:string)  [unwired: 14 in]
          }
          event "偏移值补偿": Value Change {
            n145 = event-data() -> ("NewVal"=w273:dbl)  [unwired: 1 in, 5 out]
            n146 = global read "多参数全局变量.vi" "MB session in"() -> (w275:refnum<class "MB_Master.lvclass">)
            n147 = call "000CH_电导率_电导率偏移修正值写入.vi"("数值"=w273, "MB session in"=w275) -> ("error out"=w274:errorcluster)  [unwired: 8 in, 1 out]
            n148 = Enqueue Element At Opposite End(queue=w271, element=T1."Cond" ("元素"), error in (no error)=w274) -> (error out=w272:errorcluster)  [unwired: 1 in, 2 out]
            n149 = call "Add State to Queue.vi"("State(s) In (\"\")"=w278) -> ("States Out"=w277:string)  [unwired: 14 in]
          }
          event "温度补偿系数": Value Change {
            n150 = event-data() -> ("NewVal"=w283:dbl)  [unwired: 1 in, 5 out]
            n151 = global read "多参数全局变量.vi" "MB session in"() -> (w284:refnum<class "MB_Master.lvclass">)
            n152 = call "000AH_电导率_温度补偿系数写入.vi"("数值"=w283, "MB session in"=w284) -> ("error out"=w282:errorcluster)  [unwired: 8 in, 1 out]
            n153 = Enqueue Element At Opposite End(queue=w280, element=T1."Cond" ("元素"), error in (no error)=w282) -> (error out=w281:errorcluster)  [unwired: 1 in, 2 out]
            n154 = call "Add State to Queue.vi"("State(s) In (\"\")"=w287) -> ("States Out"=w286:string)  [unwired: 14 in]
          }
          event "刷新按钮": Value Change {
            n155 = event-data() -> ()  [unwired: 1 in, 6 out]
            n156 = call "Add State to Queue.vi"("State(s) In (\"\")"=w292) -> ("States Out"=w291:string)  [unwired: 14 in]
            n157 = Two Button Dialog(message="请再次确实是否恢复出厂设置！" ("消息")) -> (T button?=w289:bool)  [unwired: 2 in]
            n158 = case shown="真" w289 {
              frame False {
              }
              frame True {
                w293 = u16 33 items=["Factory Reset"=33] ("数值")
                n159 = global read "多参数全局变量.vi" "MB session in"() -> (w294:refnum<class "MB_Master.lvclass">)
                n160 = call "0026H_电导率_命令寄存器写入.vi"("数值"=w293, "MB session in"=w294) -> ()  [unwired: 8 in, 2 out]
              }
            }
          }
          event "校准启动": Value Change {
            n161 = event-data() -> ()  [unwired: 1 in, 6 out]
            n162 = global read "多参数全局变量.vi" "校准运行状态"() -> (w296:T6)
            n163 = Bundle By Name(cluster=w296, "Cond"=TRUE) -> (w297:T6)
            n164 = global write "多参数全局变量.vi" "校准运行状态"(w297) -> ()
            n165 = call "Add State to Queue.vi"("State(s) In (\"\")"=w301, "State(s) At Back (\"\")"="init: all\nCal: Place standard solution\n Cal: Calibration process\nidle" ("State(s) In (\"\")")) -> ("States Out"=w300:string)  [unwired: 13 in]
          }
          event "校准停止": Value Change {
            n166 = event-data() -> ()  [unwired: 1 in, 6 out]
            n167 = call "Add State to Queue.vi"("State(s) In (\"\")"="init: all\nCal: Over\nidle" ("State(s) In (\"\")")) -> ("States Out"=w303:string)  [unwired: 14 in]
          }
        }
      }
    }
  }
